vi "Version_2.0_Single_Column_Code.vi"() -> ()   [LabVIEW 2020] (continued)
                                frame True {
                                n9494 = local read "VISA Refnum in\nfor Pump"() -> (w9876:refnum<visa-resource-name>)
                                n9495 = call "HardStopCurrentProcess (SubVI).vi"("VISA Refnum in"=w9876) -> ()  [unwired: 11 in]
                                }
                                }
                                n9496 = call "ProcessCompletionWaiter (SubVI).vi"("VISA Refnum in"=w9875) -> ()  [unwired: 11 in]
                                }
                                frame #6 {
                                n9497 = local read "VISA Refnum in\nfor Pump"() -> (w9881:refnum<visa-resource-name>)
                                n9498 = local read "Volume of Syringe"() -> (w9878:dbl)
                                n9499 = call "GoToAbsolutePosition(SubVI).vi"("Absolute Volume Position in Syringe (in ul)"=0.0, "Volume of Syringe"=w9878, "Resolution of Pumping"=T2."Standard Pumping", "Flow Rate (ul/min)"=150.0, "VISA Refnum in"=w9881) -> ()  [unwired: 6 in, 1 out]
                                }
                                frame #7 {
                                n9500 = local read "Stopper that ends \nthe main loops"() -> (w9882:bool)
                                n9501 = local read "VISA Refnum in\nfor Pump"() -> (w9883:refnum<visa-resource-name>)
                                n9502 = case shown="True" w9882 {
                                frame False {
                                }
                                frame True {
                                n9503 = local read "VISA Refnum in\nfor Pump"() -> (w9884:refnum<visa-resource-name>)
                                n9504 = call "HardStopCurrentProcess (SubVI).vi"("VISA Refnum in"=w9884) -> ()  [unwired: 11 in]
                                }
                                }
                                n9505 = call "ProcessCompletionWaiter (SubVI).vi"("VISA Refnum in"=w9883) -> ()  [unwired: 11 in]
                                }
                              }
                            }
                          }
                        }
                      }
                      frame #4 {
                        n9506 = local read "VISA Refnum in\nfor Pump"() -> (w9886:refnum<visa-resource-name>)
                        n9507 = local read "Port for \nC2-Elution"() -> (w9885:string)
                        n9508 = call "PortChanger (SubVI).vi"("Port Number"=w9885, "VISA Refnum in"=w9886) -> ()  [unwired: 10 in]
                      }
                      frame #5 {
                        n9509 = local read "VISA Refnum in\nfor Pump"() -> (w9887:refnum<visa-resource-name>)
                        n9510 = call "ProcessCompletionWaiter (SubVI).vi"("VISA Refnum in"=w9887) -> ()  [unwired: 11 in]
                      }
                      frame #6 {
                        n9511 = local read "Buffer-C2 PickUp \nFlow Rate (ul/min)"() -> (w9891:dbl)
                        n9512 = local read "Buffer-C2 Pumping\nResolution"() -> (w9890:T2)
                        n9513 = local read "VISA Refnum in\nfor Pump"() -> (w9893:refnum<visa-resource-name>)
                        n9514 = local read "Buffer-C2 Volume \nto be Pumped"() -> (w9889:dbl)
                        n9515 = local read "Volume of Syringe"() -> (w9892:dbl)
                        n9516 = call "RPickUp(SubVI).vi"("Volume to be picked up"=w9889, "Volume of Syringe"=w9892, "Resolution of PickUP"=w9890, "PickUp Flow Rate (ul/min)"=w9891, "VISA Refnum in"=w9893) -> ()  [unwired: 6 in, 1 out]
                        n9517 = local write "SEC On"(TRUE ("SEC On")) -> ()
                      }
                      frame #7 {
                        n9518 = local read "Stopper that ends \nthe main loops"() -> (w9894:bool)
                        n9519 = local read "VISA Refnum in\nfor Pump"() -> (w9895:refnum<visa-resource-name>)
                        n9520 = case shown="True" w9894 {
                          frame False {
                          }
                          frame True {
                            n9521 = local read "VISA Refnum in\nfor Pump"() -> (w9896:refnum<visa-resource-name>)
                            n9522 = call "HardStopCurrentProcess (SubVI).vi"("VISA Refnum in"=w9896) -> ()  [unwired: 11 in]
                          }
                        }
                        n9523 = call "ProcessCompletionWaiter (SubVI).vi"("VISA Refnum in"=w9895) -> ()  [unwired: 11 in]
                      }
                      frame #8 {
                        # "Reads the initial Plunger Position for computing the volume dispensed"
                        n9524 = local read "VISA Refnum in\nfor Pump"() -> (w9898:refnum<visa-resource-name>)
                        n9525 = call "AbsolutePlungerPosition (SubVI).vi"("VISA Refnum in"=w9898) -> ("Plunger Position"=w9897:i32)  [unwired: 10 in]
                        n9526 = local write "Initial Plunger Position"(w9897) -> ()
                      }
                      frame #9 {
                        # "Switch to Port-10"
                        # "Port-10 of the pump is conncted to column-2 of chip"
                        n9527 = local read "VISA Refnum in\nfor Pump"() -> (w9900:refnum<visa-resource-name>)
                        n9528 = call "PortChanger (SubVI).vi"("Port Number"="10", "VISA Refnum in"=w9900) -> ()  [unwired: 10 in]
                      }
                      frame #10 {
                        n9529 = local read "Stopper that ends \nthe main loops"() -> (w9901:bool)
                        n9530 = local read "VISA Refnum in\nfor Pump"() -> (w9902:refnum<visa-resource-name>)
                        n9531 = call "ProcessCompletionWaiter (SubVI).vi"("VISA Refnum in"=w9902) -> ()  [unwired: 11 in]
                        n9532 = case shown="True" w9901 {
                          frame False {
                          }
                          frame True {
                            n9533 = local read "VISA Refnum in\nfor Pump"() -> (w9903:refnum<visa-resource-name>)
                            n9534 = call "HardStopCurrentProcess (SubVI).vi"("VISA Refnum in"=w9903) -> ()  [unwired: 11 in]
                          }
                        }
                      }
                      frame #11 {
                        # "Keeps the AMF valve after column-1 open and valve after column-2 closed"
                        n9535 = local read "Buffer-C2 Dispense\nFlow Rate (ul/min)"() -> (w9916:dbl)
                        n9536 = local read "Buffer-C2 Pumping\nResolution"() -> (w9915:T2)
                        n9537 = local read "VISA Refnum in\nfor Pump"() -> (w9918:refnum<visa-resource-name>)
                        n9538 = local write "Pause Data Collection"(FALSE ("Pause Data Collection")) -> ()
                        n9539 = local read "Volume of Syringe"() -> (w9917:dbl)
                        n9540 = call "GoToAbsolutePosition(SubVI).vi"("Absolute Volume Position in Syringe (in ul)"=0.0 ("Volume to be Dispensed"), "Volume of Syringe"=w9917, "Resolution of Pumping"=w9915, "Flow Rate (ul/min)"=w9916, "VISA Refnum in"=w9918) -> ()  [unwired: 6 in, 1 out]
                        n9541 = local write "Valve V1 Open"(FALSE ("Valve V1 Open")) -> ()
                        n9542 = local write "Valve V2 Open"(TRUE ("Valve V2 Open")) -> ()
                        n9543 = local write "Valve V3 Open"(TRUE ("Valve V3 Open")) -> ()
                        n9544 = local write "Valve V4 Open"(FALSE ("Valve V4 Open")) -> ()
                        n9545 = local write "External Valve \nOpen"(TRUE ("External Valve \nOpen")) -> ()
                        n9546 = local write "Valve V8 Open"(FALSE ("Valve V8 Open")) -> ()
                        n9547 = local write "Valve V5 Open"(FALSE ("Valve V5 Open")) -> ()
                        n9548 = local write "Valve V6 Open"(FALSE ("Valve V6 Open")) -> ()
                        n9549 = local write "Valve V7 Open"(FALSE ("Valve V7 Open")) -> ()
                      }
                      frame #12 {
                        n9550 = local read "Initial Plunger Position"() -> (w9922:dbl)
                        n9551 = local read "Buffer-C2 Pumping\nResolution"() -> (w9921:T2)
                        n9552 = local read "VISA Refnum in\nfor Pump"() -> (w9923:refnum<visa-resource-name>)
                        n9553 = local read "Volume of Syringe"() -> (w9920:dbl)
                        n9554 = while {
                          tunnel: w9922 -> [w9929]
                          tunnel: w9923 -> [w9928]
                          tunnel: w9921 -> [w9927]
                          tunnel: w9920 -> [w9926]
                          stop <- w9924 stop-if-true
                          n9555 = Wait (ms)(milliseconds to wait=u32 100) -> ()  [unwired: 1 out]
                          n9556 = stacked-sequence {
                            tunnel: w9929 -> [w9935 _]
                            tunnel: w9928 -> [w9934 w9961]
                            tunnel: w9927 -> [w9933 _]
                            tunnel: w9926 -> [w9932 _]
                            tunnel: [_ w9957] -> w9924
                            frame #0 {
                              n9557 = call "AbsolutePlungerPosition (SubVI).vi"("VISA Refnum in"=w9934) -> ("Plunger Position"=w9931:i32)  [unwired: 10 in]
                              n9558 = case shown="\"Standard Pumping\", Default" w9933 {
                                tunnel: w9935 -> [w9940 w9949]
                                tunnel: w9931 -> [w9941 w9948]
                                tunnel: [w9939 w9946] -> w9930
                                tunnel: w9932 -> [w9938 w9947]
                                frame "Standard Pumping", Default {
                                n9559 = Subtract(x=w9940, y=w9941) -> (x-y=w9937:dbl)
                                n9560 = Absolute Value(x=w9937) -> (abs(x)=w9936:dbl)
                                n9561 = Multiply(x=w9936, y=w9938) -> (x*y=w9943:dbl)
                                n9562 = Divide(x=w9943, y=3000.0) -> (x/y=w9939:dbl)
                                }
                                frame "High Resolution Pumping" {
                                n9563 = Subtract(x=w9949, y=w9948) -> (x-y=w9945:dbl)
                                n9564 = Absolute Value(x=w9945) -> (abs(x)=w9944:dbl)
                                n9565 = Multiply(x=w9944, y=w9947) -> (x*y=w9951:dbl)
                                n9566 = Divide(x=w9951, y=24000.0) -> (x/y=w9946:dbl)
                                }
                              }
                              n9567 = local write "Volume being Injected \nin this process"(w9930) -> ()
                            }
                            frame #1 {
                              n9568 = local read "Stopper that ends \nthe main loops"() -> (w9958:bool)
                              n9569 = local read "Divert Buffer-C \ninto Column-2"() -> (w9959:bool)
                              n9570 = local read "Volume being Injected \nin this process"() -> (w9956:dbl)
                              n9571 = call "LSPOneStatus (SubVI).vi"("VISA Refnum in"=w9961) -> ("read buffer"=w9963:string)  [unwired: 10 in]
                              n9572 = call <vilib>:"Trim Whitespace.vi"("string"=w9963) -> ("trimmed string"=w9962:string)  [unwired: 1 in]
                              n9573 = Equal?(x=w9962, y="/0`\u0003") -> (x = y?=w9960:bool)
                              n9574 = Or(x=w9959, y=w9958) -> (x .or. y?=w9954:bool)
                              n9575 = Greater Or Equal?(x=w9956, y=2.0) -> (x >= y?=w9953:bool)
                              n9576 = Or(x=w9954, y=w9953) -> (x .or. y?=w9952:bool)
                              n9577 = Or(x=w9960, y=w9952) -> (x .or. y?=w9957:bool)
                            }
                          }
                        }
                        n9578 = local read "Stopper that ends \nthe main loops"() -> (w9919:bool)
                        n9579 = case shown="True" w9919 {
                          frame False {
                          }
                          frame True {
                            n9580 = local read "VISA Refnum in\nfor Pump"() -> (w9965:refnum<visa-resource-name>)
                            n9581 = call "HardStopCurrentProcess (SubVI).vi"("VISA Refnum in"=w9965) -> ()  [unwired: 11 in]
                          }
                        }
                      }
                      frame #13 {
                        # "Keeps the on-chip valves V4, V5 and V7 open"
                        # "Keeps the AMF valve after column-1 closed and valve after column-2 open"
                        n9582 = local write "Divert Buffer-C \ninto Column-2"(FALSE ("Divert Buffer-C \ninto Column-2")) -> ()
                        n9583 = local write "Valve V3 Open"(TRUE ("Valve V3 Open")) -> ()
                        n9584 = local write "Valve V2 Open"(FALSE ("Valve V2 Open")) -> ()
                        n9585 = local write "Valve V1 Open"(FALSE ("Valve V1 Open")) -> ()
                        n9586 = local write "Valve V4 Open"(TRUE ("Valve V4 Open")) -> ()
                        n9587 = local write "External Valve \nOpen"(FALSE ("External Valve \nOpen")) -> ()
                        n9588 = local write "Valve V5 Open"(TRUE ("Valve V5 Open")) -> ()
                        n9589 = local write "Valve V6 Open"(FALSE ("Valve V6 Open")) -> ()
                        n9590 = local write "Valve V8 Open"(FALSE ("Valve V8 Open")) -> ()
                        n9591 = local write "Valve V7 Open"(TRUE ("Valve V7 Open")) -> ()
                      }
                      frame #14 {
                        n9592 = local read "Initial Plunger Position"() -> (w9979:dbl)
                        n9593 = local read "Buffer-C2 Pumping\nResolution"() -> (w9978:T2)
                        n9594 = local read "VISA Refnum in\nfor Pump"() -> (w9980:refnum<visa-resource-name>)
                        n9595 = local read "Volume of Syringe"() -> (w9977:dbl)
                        n9596 = while {
                          tunnel: w9979 -> [w9986]
                          tunnel: w9980 -> [w9985]
                          tunnel: w9978 -> [w9984]
                          tunnel: w9977 -> [w9983]
                          stop <- w9981 stop-if-true
                          n9597 = Wait (ms)(milliseconds to wait=u32 100) -> ()  [unwired: 1 out]
                          n9598 = stacked-sequence {
                            tunnel: w9986 -> [w9992 _]
                            tunnel: w9985 -> [w9991 w10014]
                            tunnel: w9984 -> [w9990 _]
                            tunnel: w9983 -> [w9989 _]
                            tunnel: [_ w10012] -> w9981
                            frame #0 {
                              n9599 = call "AbsolutePlungerPosition (SubVI).vi"("VISA Refnum in"=w9991) -> ("Plunger Position"=w9988:i32)  [unwired: 10 in]
                              n9600 = case shown="\"Standard Pumping\", Default" w9990 {
                                tunnel: w9992 -> [w9997 w10006]
                                tunnel: w9988 -> [w9998 w10005]
                                tunnel: [w9996 w10003] -> w9987
                                tunnel: w9989 -> [w9995 w10004]
                                frame "Standard Pumping", Default {
                                n9601 = Subtract(x=w9997, y=w9998) -> (x-y=w9994:dbl)
                                n9602 = Absolute Value(x=w9994) -> (abs(x)=w9993:dbl)
                                n9603 = Multiply(x=w9993, y=w9995) -> (x*y=w10000:dbl)
                                n9604 = Divide(x=w10000, y=3000.0) -> (x/y=w9996:dbl)
                                }
                                frame "High Resolution Pumping" {
                                n9605 = Subtract(x=w10006, y=w10005) -> (x-y=w10002:dbl)
                                n9606 = Absolute Value(x=w10002) -> (abs(x)=w10001:dbl)
                                n9607 = Multiply(x=w10001, y=w10004) -> (x*y=w10008:dbl)
                                n9608 = Divide(x=w10008, y=24000.0) -> (x/y=w10003:dbl)
                                }
                              }
                              n9609 = local write "Volume being Injected \nin this process"(w9987) -> ()
                            }
                            frame #1 {
                              n9610 = call "LSPOneStatus (SubVI).vi"("VISA Refnum in"=w10014) -> ("read buffer"=w10016:string)  [unwired: 10 in]
                              n9611 = call <vilib>:"Trim Whitespace.vi"("string"=w10016) -> ("trimmed string"=w10015:string)  [unwired: 1 in]
                              n9612 = Equal?(x=w10015, y="/0`\u0003") -> (x = y?=w10013:bool)
                              n9613 = local read "Stopper that ends \nthe main loops"() -> (w10010:bool)
                              n9614 = local read "Divert Sample \nonto Grid"() -> (w10011:bool)
                              n9615 = Or(x=w10011, y=w10010) -> (x .or. y?=w10009:bool)
                              n9616 = Or(x=w10013, y=w10009) -> (x .or. y?=w10012:bool)
                            }
                          }
                        }
                        n9617 = local read "Stopper that ends \nthe main loops"() -> (w9976:bool)
                        n9618 = case shown="True" w9976 {
                          frame False {
                          }
                          frame True {
                            n9619 = local read "VISA Refnum in\nfor Pump"() -> (w10018:refnum<visa-resource-name>)
                            n9620 = call "HardStopCurrentProcess (SubVI).vi"("VISA Refnum in"=w10018) -> ()  [unwired: 11 in]
                          }
                        }
                      }
                      frame #15 {
                        n9621 = local read "Volume being Injected \nin this process"() -> (w10021:dbl)
                        n9622 = local read "VISA Refnum in\nfor Pump"() -> (w10023:refnum<visa-resource-name>)
                        n9623 = call "AbsolutePlungerPosition (SubVI).vi"("VISA Refnum in"=w10023) -> ("Plunger Position"=w10022:i32)  [unwired: 10 in]
                        n9624 = local write "Pause Data Collection"(TRUE) -> ()
                        n9625 = local write "True Volume being \ninjected in this\nprocess"(w10021) -> ()
                        n9626 = local write "Position\nNow"(w10022) -> ()
                        n9627 = Wait (ms)(milliseconds to wait=u32 500) -> ()  [unwired: 1 out]
                      }
                      frame #16 {
                        # "Sample Deposition onto EM-Grid"
                        n9628 = local read "Divert Sample \nonto Grid"() -> (w10024:bool)
                        n9629 = case shown="True" w10024 {
                          frame False {
                          }
                          frame True {
                            n9630 = stacked-sequence {
                              frame #0 {
                                # "Discard the initial volume of fluid that is present in the channel prior to detection"
                                n9631 = local read "Buffer-C2 Pumping\nResolution"() -> (w10037:T2)
                                n9632 = local read "Initial Plunger Position"() -> (w10036:dbl)
                                n9633 = local read "VISA Refnum in\nfor Pump"() -> (w10038:refnum<visa-resource-name>)
                                n9634 = local read "Position\nNow"() -> (w10034:dbl)
                                n9635 = local read "Volume of Syringe"() -> (w10035:dbl)
                                n9636 = local write "Pause Data Collection"(FALSE) -> ()
                                n9637 = while {
                                tunnel: w10038 -> [w10048]
                                tunnel: w10037 -> [w10047]
                                tunnel: w10036 -> [w10043]
                                tunnel: w10035 -> [w10046]
                                tunnel: w10034 -> [w10042]
                                stop <- w10044 stop-if-true
                                n9638 = stacked-sequence {
                                tunnel: w10048 -> [w10054 w10076 w10108]
                                tunnel: w10047 -> [w10053 w10075 _]
                                tunnel: w10043 -> [w10051 _ _]
                                tunnel: w10046 -> [w10050 w10073 _]
                                tunnel: [_ _ w10102] -> w10044
                                tunnel: w10042 -> [_ w10071 _]
                                frame #0 {
                                # "From here on 'True Volume being injected \nin this process' represents the true total \nvolume in this process"
                                n9639 = call "AbsolutePlungerPosition (SubVI).vi"("VISA Refnum in"=w10054) -> ("Plunger Position"=w10052:i32)  [unwired: 10 in]
                                n9640 = case shown="..\"Standard Pumping\"" w10053 {
                                tunnel: w10052 -> [w10062 w10070]
                                tunnel: w10051 -> [w10061 w10069]
                                tunnel: w10050 -> [w10058 w10066]
                                tunnel: [w10055 w10063] -> w10049
                                frame .."Standard Pumping" {
                                n9641 = Subtract(x=w10062, y=w10061) -> (x-y=w10060:dbl)
                                n9642 = Absolute Value(x=w10060) -> (abs(x)=w10059:dbl)
                                n9643 = Multiply(x=w10059, y=w10058) -> (x*y=w10057:dbl)
                                n9644 = Divide(x=w10057, y=3000.0) -> (x/y=w10055:dbl)
                                }
                                frame "High Resolution Pumping".. {
                                n9645 = Subtract(x=w10070, y=w10069) -> (x-y=w10068:dbl)
                                n9646 = Absolute Value(x=w10068) -> (abs(x)=w10067:dbl)
                                n9647 = Multiply(x=w10067, y=w10066) -> (x*y=w10065:dbl)
                                n9648 = Divide(x=w10065, y=24000.0) -> (x/y=w10063:dbl)
                                }
                                }
                                n9649 = local write "True Volume being \ninjected in this\nprocess"(w10049) -> ()
                                }
                                frame #1 {
                                # "From here on 'Volume being injected \nin this process' represents the volume \nin this sub process"
                                n9650 = call "AbsolutePlungerPosition (SubVI).vi"("VISA Refnum in"=w10076) -> ("Plunger Position"=w10074:i32)  [unwired: 10 in]
                                n9651 = case shown="..\"Standard Pumping\"" w10075 {
                                tunnel: w10074 -> [w10084 w10092]
                                tunnel: w10071 -> [w10083 w10091]
                                tunnel: w10073 -> [w10080 w10088]
                                tunnel: [w10077 w10085] -> w10072
                                frame .."Standard Pumping" {
                                n9652 = Subtract(x=w10084, y=w10083) -> (x-y=w10082:dbl)
                                n9653 = Absolute Value(x=w10082) -> (abs(x)=w10081:dbl)
                                n9654 = Multiply(x=w10081, y=w10080) -> (x*y=w10079:dbl)
                                n9655 = Divide(x=w10079, y=3000.0) -> (x/y=w10077:dbl)
                                }
                                frame "High Resolution Pumping".. {
                                n9656 = Subtract(x=w10092, y=w10091) -> (x-y=w10090:dbl)
                                n9657 = Absolute Value(x=w10090) -> (abs(x)=w10089:dbl)
                                n9658 = Multiply(x=w10089, y=w10088) -> (x*y=w10087:dbl)
                                n9659 = Divide(x=w10087, y=24000.0) -> (x/y=w10085:dbl)
                                }
                                }
                                n9660 = local write "Volume being Injected \nin this process"(w10072) -> ()
                                }
                                frame #2 {
                                n9661 = local read "Discard Volume"() -> (w10096:dbl)
                                n9662 = local read "Discard fluid \nprior to 1st \ndeposition"() -> (w10101:bool)
                                n9663 = local read "Volume being Injected \nin this process"() -> (w10100:dbl)
                                n9664 = Greater Or Equal?(x=w10100, y=w10096) -> (x >= y?=w10098:bool)
                                n9665 = call "AbsolutePlungerPositionStatus (SubVI).vi"("VISA Refnum in"=w10108) -> ("read buffer"=w10107:string)  [unwired: 10 in]
                                n9666 = local read "Stop for End of \nExperiment \nand Data Writing"() -> (w10095:bool)
                                n9667 = call <vilib>:"Trim Whitespace.vi"("string"=w10107) -> ("trimmed string"=w10106:string)  [unwired: 1 in]
                                n9668 = Not(x=w10101) -> (.not. x?=w10099:bool)
                                n9669 = Equal?(x=w10106, y="/0`\u0003") -> (x = y?=w10104:bool)
                                n9670 = Or(x=w10099, y=w10098) -> (x .or. y?=w10097:bool)
                                n9671 = local read "Re-SEC"() -> (w10094:bool)
                                n9672 = Or(x=w10095, y=w10094) -> (x .or. y?=w10093:bool)
                                n9673 = Or(x=w10097, y=w10093) -> (x .or. y?=w10103:bool)
                                n9674 = Or(x=w10104, y=w10103) -> (x .or. y?=w10102:bool)
                                }
                                }
                                n9675 = Wait (ms)(milliseconds to wait=u32 100) -> ()  [unwired: 1 out]
                                }
                                n9676 = local write "Valve V4 Open"(TRUE ("Valve V4 Open")) -> ()
                                n9677 = local write "Valve V3 Open"(TRUE ("Valve V3 Open")) -> ()
                                n9678 = local write "Valve V2 Open"(FALSE ("Valve V2 Open")) -> ()
                                n9679 = local write "Valve V1 Open"(FALSE ("Valve V1 Open")) -> ()
                                n9680 = local write "External Valve \nOpen"(FALSE ("External Valve \nOpen")) -> ()
                                n9681 = local write "Valve V5 Open"(TRUE ("Valve V5 Open")) -> ()
                                n9682 = local write "Valve V6 Open"(TRUE ("Valve V6 Open")) -> ()
                                n9683 = local write "Valve V8 Open"(FALSE ("Valve V8 Open")) -> ()
                                n9684 = local write "Valve V7 Open"(FALSE ("Valve V7 Open")) -> ()
                                n9685 = local write "Volume being Injected \nin this process"(0.0) -> ()
                              }
                              frame #1 {
                                # "Keeps the on-chip valve V1, V2 and V3 closed,\nHalts also deposition onto the grid\nand waits for the 1st redeposit command. Once the command is issued\nit starts pumpoing and moves onto the next frame"
                                n9686 = stacked-sequence {
                                frame #0 {
                                n9687 = local write "Valve V5 Open"(FALSE ("Valve V5 Open")) -> ()
                                n9688 = local write "Valve V1 Open"(FALSE ("Valve V1 Open")) -> ()
                                n9689 = local read "VISA Refnum in\nfor Pump"() -> (w10120:refnum<visa-resource-name>)
                                n9690 = local write "Valve V2 Open"(FALSE ("Valve V2 Open")) -> ()
                                n9691 = local write "Valve V6 Open"(FALSE ("Valve V6 Open")) -> ()
                                n9692 = local write "Re-deposit Sample\nonto Grid"(FALSE ("Redeposit Sample\nonto Grid")) -> ()
                                n9693 = local write "Pause Data Collection"(TRUE ("Pause Data Collection")) -> ()
                                n9694 = call "HardStopCurrentProcess (SubVI).vi"("VISA Refnum in"=w10120) -> ()  [unwired: 11 in]
                                n9695 = local write "Valve V7 Open"(FALSE ("Valve V7 Open")) -> ()
                                n9696 = local write "Valve V3 Open"(FALSE ("Valve V3 Open")) -> ()
                                n9697 = local write "External Valve \nOpen"(FALSE ("External Valve \nOpen")) -> ()
                                n9698 = local write "Valve V4 Open"(FALSE ("Valve V4 Open")) -> ()
                                n9699 = local write "Valve V8 Open"(FALSE ("Valve V8 Open")) -> ()
                                }
                                frame #1 {
                                n9700 = while {
                                stop <- w10126 stop-if-true
                                n9701 = local read "Stop for End of \nExperiment \nand Data Writing"() -> (w10124:bool)
                                n9702 = local read "Re-SEC"() -> (w10125:bool)
                                n9703 = local read "Re-deposit Sample\nonto Grid"() -> (w10127:bool)
                                n9704 = Or(x=w10124, y=w10125) -> (x .or. y?=w10123:bool)
                                n9705 = Or(x=w10127, y=w10123) -> (x .or. y?=w10126:bool)
                                }
                                n9706 = local write "Discard fluid \nprior to 1st \ndeposition"(FALSE ("Discard fluid \nprior to 1st \ndeposition")) -> ()
                                n9707 = One Button Dialog(message="Do you want to deposit sample on another grid? If yes, turn on 'Re-deposit Sample onto Grid'. Else turn on Re-SEC to do SEC again or STOP to end the experiment") -> ()  [unwired: 1 in, 1 out]
                                }
                                frame #2 {
                                n9708 = local write "Valve V6 Open"(TRUE ("Valve V3 Open")) -> ()
                                n9709 = local write "Valve V4 Open"(TRUE ("Valve V1 Open")) -> ()
                                n9710 = local write "Valve V5 Open"(TRUE ("Valve V2 Open")) -> ()
                                n9711 = local write "Valve V3 Open"(TRUE ("Valve V3 Open")) -> ()
                                n9712 = local write "Valve V7 Open"(FALSE ("Valve V7 Open")) -> ()
                                }
                                frame #3 {
                                n9713 = local read "Re-deposit Sample\nonto Grid"() -> (w10133:bool)
                                n9714 = case shown="True" w10133 {
                                frame False {
                                n9715 = local write "Suction On/Off"(FALSE ("Suction On/Off")) -> ()
                                }
                                frame True {
                                n9716 = stacked-sequence {
                                frame #0 {
                                n9717 = local read "VISA Refnum in\nfor Pump"() -> (w10136:refnum<visa-resource-name>)
                                n9718 = call "AbsolutePlungerPosition (SubVI).vi"("VISA Refnum in"=w10136) -> ("Plunger Position"=w10135:i32)  [unwired: 10 in]
                                n9719 = local write "Position\nNow"(w10135) -> ()
                                }
                                frame #1 {
                                n9720 = local read "Buffer-C2 Pumping\nResolution"() -> (w10138:T2)
                                n9721 = case shown="\"Standard Pumping\", Default" w10138 {
                                tunnel: [w10139 w10150] -> w10137
                                frame "Standard Pumping", Default {
                                n9722 = local read "Buffer-C2 Volume \nto be Pumped"() -> (w10142:dbl)
                                n9723 = local read "Volume of Syringe"() -> (w10145:dbl)
                                n9724 = local read "Initial Plunger Position"() -> (w10149:dbl)
                                n9725 = local read "Position\nNow"() -> (w10148:dbl)
                                n9726 = Subtract(x=w10149, y=w10148) -> (x-y=w10147:dbl)
                                n9727 = Absolute Value(x=w10147) -> (abs(x)=w10146:dbl)
                                n9728 = Multiply(x=w10146, y=w10145) -> (x*y=w10144:dbl)
                                n9729 = Divide(x=w10144, y=3000.0) -> (x/y=w10141:dbl)
                                n9730 = Subtract(x=w10141, y=w10142) -> (x-y=w10140:dbl)
                                n9731 = Absolute Value(x=w10140) -> (abs(x)=w10139:dbl)
                                }
                                frame "High Resolution Pumping" {
                                n9732 = local read "Buffer-C2 Volume \nto be Pumped"() -> (w10153:dbl)
                                n9733 = local read "Volume of Syringe"() -> (w10156:dbl)
                                n9734 = local read "Initial Plunger Position"() -> (w10160:dbl)
                                n9735 = local read "Position\nNow"() -> (w10159:dbl)
                                n9736 = Subtract(x=w10160, y=w10159) -> (x-y=w10158:dbl)
                                n9737 = Absolute Value(x=w10158) -> (abs(x)=w10157:dbl)
                                n9738 = Multiply(x=w10157, y=w10156) -> (x*y=w10155:dbl)
                                n9739 = Divide(x=w10155, y=24000.0) -> (x/y=w10152:dbl)
                                n9740 = Subtract(x=w10152, y=w10153) -> (x-y=w10151:dbl)
                                n9741 = Absolute Value(x=w10151) -> (abs(x)=w10150:dbl)
                                }
                                }
                                n9742 = local write "Buffer-C Volume\nleft to be Pumped"(w10137) -> ()
                                }
                                frame #2 {
                                n9743 = local read "Buffer-C2 Dispense\nFlow Rate (ul/min)"() -> (w10164:dbl)
                                n9744 = local read "Buffer-C2 Pumping\nResolution"() -> (w10163:T2)
                                n9745 = local read "VISA Refnum in\nfor Pump"() -> (w10166:refnum<visa-resource-name>)
                                n9746 = local read "Volume of Syringe"() -> (w10165:dbl)
                                n9747 = call "GoToAbsolutePosition(SubVI).vi"("Absolute Volume Position in Syringe (in ul)"=0.0, "Volume of Syringe"=w10165, "Resolution of Pumping"=w10163, "Flow Rate (ul/min)"=w10164, "VISA Refnum in"=w10166) -> ()  [unwired: 6 in, 1 out]
                                n9748 = local write "Suction On/Off"(FALSE ("Suction On/Off")) -> ()
                                }
                                }
                                }
                                }
                                }
                                frame #4 {
                                n9749 = local read "Stop for End of \nExperiment \nand Data Writing"() -> (w10169:bool)
                                n9750 = local read "Re-SEC"() -> (w10168:bool)
                                n9751 = Or(x=w10169, y=w10168) -> (x .or. y?=w10167:bool)
                                n9752 = case shown="True" w10167 {
                                frame False {
                                }
                                frame True {
                                n9753 = local read "VISA Refnum in\nfor Pump"() -> (w10170:refnum<visa-resource-name>)
                                n9754 = call "HardStopCurrentProcess (SubVI).vi"("VISA Refnum in"=w10170) -> ()  [unwired: 11 in]
                                }
                                }
                                }
                                }
                              }
                              frame #2 {
                                # "Keeps the on-chip valve V1, V2 Open and V3 closed"
                                n9755 = while {
                                stop <- w10176 stop-if-true
                                n9756 = local read "Suction On/Off"() -> (w10177:bool)
                                n9757 = case shown="True" w10177 {
                                frame False {
                                n9758 = local read "Buffer-C2 Pumping\nResolution"() -> (w10183:T2)
                                n9759 = local read "Initial Plunger Position"() -> (w10182:dbl)
                                n9760 = local read "VISA Refnum in\nfor Pump"() -> (w10184:refnum<visa-resource-name>)
                                n9761 = local read "Position\nNow"() -> (w10180:dbl)
                                n9762 = local read "Volume of Syringe"() -> (w10181:dbl)
                                n9763 = local write "Volume being Injected \nin this process"(0.0) -> ()
                                n9764 = local write "Pause Data Collection"(FALSE) -> ()
                                n9765 = while {
                                tunnel: w10184 -> [w10191]
                                tunnel: w10183 -> [w10190]
                                tunnel: w10182 -> [w10186]
                                tunnel: w10181 -> [w10189]
                                tunnel: w10180 -> [w10185]
                                stop <- w10187 stop-if-true
                                n9766 = stacked-sequence {
                                tunnel: w10191 -> [w10197 w10219 w10246]
                                tunnel: w10190 -> [w10196 w10218 _]
                                tunnel: w10186 -> [w10194 _ _]
                                tunnel: w10189 -> [w10193 w10216 _]
                                tunnel: [_ _ w10239] -> w10187
                                tunnel: w10185 -> [_ w10214 _]
                                frame #0 {
                                # "From here on 'True Volume being injected \nin this process' represents the true total \nvolume in this process"
                                n9767 = call "AbsolutePlungerPosition (SubVI).vi"("VISA Refnum in"=w10197) -> ("Plunger Position"=w10195:i32)  [unwired: 10 in]
                                n9768 = case shown="..\"Standard Pumping\"" w10196 {
                                tunnel: w10195 -> [w10205 w10213]
                                tunnel: w10194 -> [w10204 w10212]
                                tunnel: w10193 -> [w10201 w10209]
                                tunnel: [w10198 w10206] -> w10192
                                frame .."Standard Pumping" {
                                n9769 = Subtract(x=w10205, y=w10204) -> (x-y=w10203:dbl)
                                n9770 = Absolute Value(x=w10203) -> (abs(x)=w10202:dbl)
                                n9771 = Multiply(x=w10202, y=w10201) -> (x*y=w10200:dbl)
                                n9772 = Divide(x=w10200, y=3000.0) -> (x/y=w10198:dbl)
                                }
                                frame "High Resolution Pumping".. {
                                n9773 = Subtract(x=w10213, y=w10212) -> (x-y=w10211:dbl)
                                n9774 = Absolute Value(x=w10211) -> (abs(x)=w10210:dbl)
                                n9775 = Multiply(x=w10210, y=w10209) -> (x*y=w10208:dbl)
                                n9776 = Divide(x=w10208, y=24000.0) -> (x/y=w10206:dbl)
                                }
                                }
                                n9777 = local write "True Volume being \ninjected in this\nprocess"(w10192) -> ()
                                }
                                frame #1 {
                                # "From here on 'Volume being injected \nin this process' represents the volume \nin this sub process"
                                n9778 = call "AbsolutePlungerPosition (SubVI).vi"("VISA Refnum in"=w10219) -> ("Plunger Position"=w10217:i32)  [unwired: 10 in]
                                n9779 = case shown="\"High Resolution Pumping\".." w10218 {
                                tunnel: w10217 -> [w10227 w10235]
                                tunnel: w10214 -> [w10226 w10234]
                                tunnel: w10216 -> [w10223 w10231]
                                tunnel: [w10220 w10228] -> w10215
                                frame .."Standard Pumping" {
                                n9780 = Subtract(x=w10227, y=w10226) -> (x-y=w10225:dbl)
                                n9781 = Absolute Value(x=w10225) -> (abs(x)=w10224:dbl)
                                n9782 = Multiply(x=w10224, y=w10223) -> (x*y=w10222:dbl)
                                n9783 = Divide(x=w10222, y=3000.0) -> (x/y=w10220:dbl)
                                }
                                frame "High Resolution Pumping".. {
                                n9784 = Subtract(x=w10235, y=w10234) -> (x-y=w10233:dbl)
                                n9785 = Absolute Value(x=w10233) -> (abs(x)=w10232:dbl)
                                n9786 = Multiply(x=w10232, y=w10231) -> (x*y=w10230:dbl)
                                n9787 = Divide(x=w10230, y=24000.0) -> (x/y=w10228:dbl)
                                }
                                }
                                n9788 = local write "Volume being Injected \nin this process"(w10215) -> ()
                                }
                                frame #2 {
                                n9789 = local read "Stop for End of \nExperiment \nand Data Writing"() -> (w10238:bool)
                                n9790 = local read "Re-SEC"() -> (w10237:bool)
                                n9791 = local read "Suction On/Off"() -> (w10242:bool)
                                n9792 = call "AbsolutePlungerPositionStatus (SubVI).vi"("VISA Refnum in"=w10246) -> ("read buffer"=w10245:string)  [unwired: 10 in]
                                n9793 = call <vilib>:"Trim Whitespace.vi"("string"=w10245) -> ("trimmed string"=w10244:string)  [unwired: 1 in]
                                n9794 = Equal?(x=w10244, y="/0`\u0003") -> (x = y?=w10241:bool)
                                n9795 = Or(x=w10238, y=w10237) -> (x .or. y?=w10236:bool)
                                n9796 = Or(x=w10242, y=w10236) -> (x .or. y?=w10240:bool)
                                n9797 = Or(x=w10241, y=w10240) -> (x .or. y?=w10239:bool)
                                }
                                }
                                n9798 = Wait (ms)(milliseconds to wait=u32 100) -> ()  [unwired: 1 out]
                                }
                                }
                                frame True {
                                n9799 = stacked-sequence {
                                frame #0 {
                                n9800 = local write "Valve V3 Open"(FALSE ("Valve V3 Open")) -> ()
                                n9801 = local read "Suction Pressure\nfor EM-grid \nDeposition (mbar)"() -> (w10253:sgl)
                                n9802 = local write "Valve V4 Open"(FALSE ("Valve V4 Open")) -> ()
                                n9803 = local read "VISA Refnum in\nfor Pump"() -> (w10256:refnum<visa-resource-name>)
                                n9804 = local write "Valve V5 Open"(FALSE ("Valve V1 Open")) -> ()
                                n9805 = local write "Suction pressure \nfor grid deposition"(w10253) -> ()
                                n9806 = local write "Re-deposit Sample\nonto Grid"(FALSE ("Redeposit Sample\nonto Grid")) -> ()
                                n9807 = local write "Pause Data Collection"(TRUE ("Pause Data Collection")) -> ()
                                n9808 = call "HardStopCurrentProcess (SubVI).vi"("VISA Refnum in"=w10256) -> ()  [unwired: 11 in]
                                n9809 = local write "Valve V6 Open"(TRUE ("Valve V2 Open")) -> ()
                                n9810 = local write "Valve V7 Open"(TRUE ("Valve V3 Open")) -> ()
                                n9811 = local write "External Valve \nOpen"(FALSE ("External Valve \nOpen")) -> ()
                                }
                                frame #1 {
                                n9812 = while {
                                stop <- w10259 stop-if-true
                                n9813 = local read "Stop for End of \nExperiment \nand Data Writing"() -> (w10260:bool)
                                n9814 = local read "Suction Pressure\nfor EM-grid \nDeposition (mbar)"() -> (w10257:sgl)
                                n9815 = call <vilib>:"fgt set pressure.vi"("pressure"=w10257, "pressureIndex"=u32 1) -> ()  [unwired: 9 in, 1 out]
                                n9816 = local read "Suction On/Off"() -> (w10262:bool)
                                n9817 = Not(x=w10262) -> (.not. x?=w10261:bool)
                                n9818 = Wait (ms)(milliseconds to wait=u32 100) -> ()  [unwired: 1 out]
                                n9819 = Or(x=w10261, y=w10260) -> (x .or. y?=w10259:bool)
                                }
                                }
                                frame #2 {
                                n9820 = for {
                                N: 2 -> [_]
                                n9821 = while {
                                stop <- w10272 stop-if-true
                                n9822 = local read "Stop for End of \nExperiment \nand Data Writing"() -> (w10268:bool)
                                n9823 = local read "Suction On/Off"() -> (w10270:bool)
                                n9824 = call <vilib>:"fgt set pressure.vi"("pressure"=sgl 0.0, "pressureIndex"=u32 1) -> ()  [unwired: 9 in, 1 out]
                                n9825 = Not(x=w10270) -> (.not. x?=w10269:bool)
                                n9826 = Wait (ms)(milliseconds to wait=u32 100) -> ()  [unwired: 1 out]
                                n9827 = Or(x=w10269, y=w10268) -> (x .or. y?=w10272:bool)
                                }
                                n9828 = Wait (ms)(milliseconds to wait=u32 400) -> ()  [unwired: 1 out]
                                }
                                }
                                frame #3 {
                                n9829 = local read "Automatic purging \nof capillary after \ngrid deposition"() -> (w10273:bool)
                                n9830 = case shown="True" w10273 {
                                frame False {
                                }
                                frame True {
                                n9831 = stacked-sequence {
                                frame #0 {
                                n9832 = local read "VISA Refnum in\nfor Pump"() -> (w10275:refnum<visa-resource-name>)
                                n9833 = call "AbsolutePlungerPosition (SubVI).vi"("VISA Refnum in"=w10275) -> ("Plunger Position"=w10274:i32)  [unwired: 10 in]
                                n9834 = local write "Position\nNow"(w10274) -> ()
                                }
                                frame #1 {
                                n9835 = local read "Buffer-C2 Pumping\nResolution"() -> (w10277:T2)
                                n9836 = case shown="\"Standard Pumping\", Default" w10277 {
                                tunnel: [w10278 w10289] -> w10276
                                frame "Standard Pumping", Default {
                                n9837 = local read "Buffer-C2 Volume \nto be Pumped"() -> (w10281:dbl)
                                n9838 = local read "Volume of Syringe"() -> (w10284:dbl)
                                n9839 = local read "Initial Plunger Position"() -> (w10288:dbl)
                                n9840 = local read "Position\nNow"() -> (w10287:dbl)
                                n9841 = Subtract(x=w10288, y=w10287) -> (x-y=w10286:dbl)
                                n9842 = Absolute Value(x=w10286) -> (abs(x)=w10285:dbl)
                                n9843 = Multiply(x=w10285, y=w10284) -> (x*y=w10283:dbl)
                                n9844 = Divide(x=w10283, y=3000.0) -> (x/y=w10280:dbl)
                                n9845 = Subtract(x=w10280, y=w10281) -> (x-y=w10279:dbl)
                                n9846 = Absolute Value(x=w10279) -> (abs(x)=w10278:dbl)
                                }
                                frame "High Resolution Pumping" {
                                n9847 = local read "Buffer-C2 Volume \nto be Pumped"() -> (w10292:dbl)
                                n9848 = local read "Volume of Syringe"() -> (w10295:dbl)
                                n9849 = local read "Initial Plunger Position"() -> (w10299:dbl)
                                n9850 = local read "Position\nNow"() -> (w10298:dbl)
                                n9851 = Subtract(x=w10299, y=w10298) -> (x-y=w10297:dbl)
                                n9852 = Absolute Value(x=w10297) -> (abs(x)=w10296:dbl)
                                n9853 = Multiply(x=w10296, y=w10295) -> (x*y=w10294:dbl)
                                n9854 = Divide(x=w10294, y=24000.0) -> (x/y=w10291:dbl)
                                n9855 = Subtract(x=w10291, y=w10292) -> (x-y=w10290:dbl)
                                n9856 = Absolute Value(x=w10290) -> (abs(x)=w10289:dbl)
                                }
                                }
                                n9857 = local write "Buffer-C Volume\nleft to be Pumped"(w10276) -> ()
                                }
                                frame #2 {
                                n9858 = local read "Buffer-C2 Dispense\nFlow Rate (ul/min)"() -> (w10308:dbl)
                                n9859 = local read "Buffer-C2 Pumping\nResolution"() -> (w10307:T2)
                                n9860 = local read "VISA Refnum in\nfor Pump"() -> (w10310:refnum<visa-resource-name>)
                                n9861 = local read "Volume of Syringe"() -> (w10309:dbl)
                                n9862 = call "GoToAbsolutePosition(SubVI).vi"("Absolute Volume Position in Syringe (in ul)"=0.0, "Volume of Syringe"=w10309, "Resolution of Pumping"=w10307, "Flow Rate (ul/min)"=w10308, "VISA Refnum in"=w10310) -> ()  [unwired: 6 in, 1 out]
                                n9863 = local write "External Valve \nOpen"(FALSE ("External Valve \nOpen")) -> ()
                                n9864 = local write "Valve V3 Open"(TRUE ("Valve V3 Open")) -> ()
                                n9865 = local write "Valve V7 Open"(FALSE ("Valve V3 Open")) -> ()
                                n9866 = local write "Valve V5 Open"(TRUE ("Valve V1 Open")) -> ()
                                n9867 = local write "Valve V6 Open"(TRUE ("Valve V2 Open")) -> ()
                                n9868 = local write "Valve V4 Open"(TRUE ("Valve V4 Open")) -> ()
                                }
                                frame #3 {
                                n9869 = local read "Buffer-C2 Pumping\nResolution"() -> (w10316:T2)
                                n9870 = local read "Initial Plunger Position"() -> (w10315:dbl)
                                n9871 = local read "VISA Refnum in\nfor Pump"() -> (w10317:refnum<visa-resource-name>)
                                n9872 = local read "Position\nNow"() -> (w10313:dbl)
                                n9873 = local read "Volume of Syringe"() -> (w10314:dbl)
                                n9874 = local write "Volume being Injected \nin this process"(0.0) -> ()
                                n9875 = local write "Pause Data Collection"(FALSE) -> ()
                                n9876 = while {
                                tunnel: w10317 -> [w10324]
                                tunnel: w10316 -> [w10323]
                                tunnel: w10315 -> [w10319]
                                tunnel: w10314 -> [w10322]
                                tunnel: w10313 -> [w10318]
                                stop <- w10320 stop-if-true
                                n9877 = stacked-sequence {
                                tunnel: w10324 -> [w10330 w10352 w10381]
                                tunnel: w10323 -> [w10329 w10351 _]
                                tunnel: w10319 -> [w10327 _ _]
                                tunnel: w10322 -> [w10326 w10349 _]
                                tunnel: [_ _ w10375] -> w10320
                                tunnel: w10318 -> [_ w10347 _]
                                frame #0 {
                                # "From here on 'True Volume being injected \nin this process' represents the true total \nvolume in this process"
                                n9878 = call "AbsolutePlungerPosition (SubVI).vi"("VISA Refnum in"=w10330) -> ("Plunger Position"=w10328:i32)  [unwired: 10 in]
                                n9879 = case shown="..\"Standard Pumping\"" w10329 {
                                tunnel: w10328 -> [w10338 w10346]
                                tunnel: w10327 -> [w10337 w10345]
                                tunnel: w10326 -> [w10334 w10342]
                                tunnel: [w10331 w10339] -> w10325
                                frame .."Standard Pumping" {
                                n9880 = Subtract(x=w10338, y=w10337) -> (x-y=w10336:dbl)
                                n9881 = Absolute Value(x=w10336) -> (abs(x)=w10335:dbl)
                                n9882 = Multiply(x=w10335, y=w10334) -> (x*y=w10333:dbl)
                                n9883 = Divide(x=w10333, y=3000.0) -> (x/y=w10331:dbl)
                                }
                                frame "High Resolution Pumping".. {
                                n9884 = Subtract(x=w10346, y=w10345) -> (x-y=w10344:dbl)
                                n9885 = Absolute Value(x=w10344) -> (abs(x)=w10343:dbl)
                                n9886 = Multiply(x=w10343, y=w10342) -> (x*y=w10341:dbl)
                                n9887 = Divide(x=w10341, y=24000.0) -> (x/y=w10339:dbl)
                                }
                                }
                                n9888 = local write "True Volume being \ninjected in this\nprocess"(w10325) -> ()
                                }
                                frame #1 {
                                # "From here on 'Volume being injected \nin this process' represents the volume \nin this sub process"
                                n9889 = call "AbsolutePlungerPosition (SubVI).vi"("VISA Refnum in"=w10352) -> ("Plunger Position"=w10350:i32)  [unwired: 10 in]
                                n9890 = case shown="\"High Resolution Pumping\".." w10351 {
                                tunnel: w10350 -> [w10360 w10368]
                                tunnel: w10347 -> [w10359 w10367]
                                tunnel: w10349 -> [w10356 w10364]
                                tunnel: [w10353 w10361] -> w10348
                                frame .."Standard Pumping" {
                                n9891 = Subtract(x=w10360, y=w10359) -> (x-y=w10358:dbl)
                                n9892 = Absolute Value(x=w10358) -> (abs(x)=w10357:dbl)
                                n9893 = Multiply(x=w10357, y=w10356) -> (x*y=w10355:dbl)
                                n9894 = Divide(x=w10355, y=3000.0) -> (x/y=w10353:dbl)
                                }
                                frame "High Resolution Pumping".. {
                                n9895 = Subtract(x=w10368, y=w10367) -> (x-y=w10366:dbl)
                                n9896 = Absolute Value(x=w10366) -> (abs(x)=w10365:dbl)
                                n9897 = Multiply(x=w10365, y=w10364) -> (x*y=w10363:dbl)
                                n9898 = Divide(x=w10363, y=24000.0) -> (x/y=w10361:dbl)
                                }
                                }
                                n9899 = local write "Volume being Injected \nin this process"(w10348) -> ()
                                }
                                frame #2 {
                                n9900 = local read "Capillary purge \nvolume after every\ngrid plunging"() -> (w10370:dbl)
                                n9901 = local read "Stop for End of \nExperiment \nand Data Writing"() -> (w10374:bool)
                                n9902 = local read "Volume being Injected \nin this process"() -> (w10371:dbl)
                                n9903 = local read "Re-SEC"() -> (w10373:bool)
                                n9904 = call "AbsolutePlungerPositionStatus (SubVI).vi"("VISA Refnum in"=w10381) -> ("read buffer"=w10380:string)  [unwired: 10 in]
                                n9905 = call <vilib>:"Trim Whitespace.vi"("string"=w10380) -> ("trimmed string"=w10379:string)  [unwired: 1 in]
                                n9906 = Greater Or Equal?(x=w10371, y=w10370) -> (x >= y?=w10369:bool)
                                n9907 = Equal?(x=w10379, y="/0`\u0003") -> (x = y?=w10377:bool)
                                n9908 = Or(x=w10374, y=w10373) -> (x .or. y?=w10372:bool)
                                n9909 = Or(x=w10369, y=w10372) -> (x .or. y?=w10376:bool)
                                n9910 = Or(x=w10377, y=w10376) -> (x .or. y?=w10375:bool)
                                }
                                }
                                n9911 = Wait (ms)(milliseconds to wait=u32 100) -> ()  [unwired: 1 out]
                                }
                                }
                                frame #4 {
                                n9912 = local read "VISA Refnum in\nfor Pump"() -> (w10382:refnum<visa-resource-name>)
                                n9913 = call "HardStopCurrentProcess (SubVI).vi"("VISA Refnum in"=w10382) -> ()  [unwired: 11 in]
                                }
                                }
                                }
                                }
                                }
                                frame #4 {
                                n9914 = local write "Valve V3 Open"(FALSE ("Valve V3 Open")) -> ()
                                n9915 = local write "Valve V7 Open"(FALSE ("Valve V3 Open")) -> ()
                                n9916 = local write "Valve V5 Open"(FALSE ("Valve V1 Open")) -> ()
                                n9917 = local write "Valve V6 Open"(FALSE ("Valve V2 Open")) -> ()
                                n9918 = local write "Valve V4 Open"(FALSE ("Valve V4 Open")) -> ()
                                }
                                frame #5 {
                                n9919 = while {
                                stop <- w10392 stop-if-true
                                n9920 = local read "Stop for End of \nExperiment \nand Data Writing"() -> (w10390:bool)
                                n9921 = local read "Re-deposit Sample\nonto Grid"() -> (w10393:bool)
                                n9922 = local read "Re-SEC"() -> (w10391:bool)
                                n9923 = Or(x=w10390, y=w10391) -> (x .or. y?=w10389:bool)
                                n9924 = Or(x=w10393, y=w10389) -> (x .or. y?=w10392:bool)
                                }
                                n9925 = One Button Dialog(message="Do you want to deposit sample on another grid? If yes, turn on 'Re-deposit Sample onto Grid'. Else turn on Re-SEC to do SEC again or STOP to end the experiment") -> ()  [unwired: 1 in, 1 out]
                                }
                                frame #6 {
                                n9926 = local write "Valve V4 Open"(TRUE ("Valve V4 Open")) -> ()
                                n9927 = local write "Valve V3 Open"(TRUE ("Valve V3 Open")) -> ()
                                n9928 = local write "Valve V7 Open"(FALSE ("Valve V3 Open")) -> ()
                                n9929 = local write "Valve V5 Open"(TRUE ("Valve V1 Open")) -> ()
                                n9930 = local write "Valve V6 Open"(TRUE ("Valve V2 Open")) -> ()
                                }
                                frame #7 {
                                n9931 = local read "Re-deposit Sample\nonto Grid"() -> (w10399:bool)
                                n9932 = case shown="True" w10399 {
                                frame False {
                                n9933 = local write "Suction On/Off"(FALSE ("Suction On/Off")) -> ()
                                }
                                frame True {
                                n9934 = stacked-sequence {
                                frame #0 {
                                n9935 = local read "VISA Refnum in\nfor Pump"() -> (w10402:refnum<visa-resource-name>)
                                n9936 = call "AbsolutePlungerPosition (SubVI).vi"("VISA Refnum in"=w10402) -> ("Plunger Position"=w10401:i32)  [unwired: 10 in]
                                n9937 = local write "Position\nNow"(w10401) -> ()
                                }
                                frame #1 {
                                n9938 = local read "Buffer-C2 Pumping\nResolution"() -> (w10404:T2)
                                n9939 = case shown="\"Standard Pumping\", Default" w10404 {
                                tunnel: [w10405 w10416] -> w10403
                                frame "Standard Pumping", Default {
                                n9940 = local read "Buffer-C2 Volume \nto be Pumped"() -> (w10408:dbl)
                                n9941 = local read "Volume of Syringe"() -> (w10411:dbl)
                                n9942 = local read "Initial Plunger Position"() -> (w10415:dbl)
                                n9943 = local read "Position\nNow"() -> (w10414:dbl)
                                n9944 = Subtract(x=w10415, y=w10414) -> (x-y=w10413:dbl)
                                n9945 = Absolute Value(x=w10413) -> (abs(x)=w10412:dbl)
                                n9946 = Multiply(x=w10412, y=w10411) -> (x*y=w10410:dbl)
                                n9947 = Divide(x=w10410, y=3000.0) -> (x/y=w10407:dbl)
                                n9948 = Subtract(x=w10407, y=w10408) -> (x-y=w10406:dbl)
                                n9949 = Absolute Value(x=w10406) -> (abs(x)=w10405:dbl)
                                }
                                frame "High Resolution Pumping" {
                                n9950 = local read "Buffer-C2 Volume \nto be Pumped"() -> (w10419:dbl)
                                n9951 = local read "Volume of Syringe"() -> (w10422:dbl)
                                n9952 = local read "Initial Plunger Position"() -> (w10426:dbl)
                                n9953 = local read "Position\nNow"() -> (w10425:dbl)
                                n9954 = Subtract(x=w10426, y=w10425) -> (x-y=w10424:dbl)
                                n9955 = Absolute Value(x=w10424) -> (abs(x)=w10423:dbl)
                                n9956 = Multiply(x=w10423, y=w10422) -> (x*y=w10421:dbl)
                                n9957 = Divide(x=w10421, y=24000.0) -> (x/y=w10418:dbl)
                                n9958 = Subtract(x=w10418, y=w10419) -> (x-y=w10417:dbl)
                                n9959 = Absolute Value(x=w10417) -> (abs(x)=w10416:dbl)
                                }
                                }
                                n9960 = local write "Buffer-C Volume\nleft to be Pumped"(w10403) -> ()
                                }
                                frame #2 {
                                n9961 = local read "Buffer-C2 Dispense\nFlow Rate (ul/min)"() -> (w10430:dbl)
                                n9962 = local read "Buffer-C2 Pumping\nResolution"() -> (w10429:T2)
                                n9963 = local read "VISA Refnum in\nfor Pump"() -> (w10432:refnum<visa-resource-name>)
                                n9964 = local read "Volume of Syringe"() -> (w10431:dbl)
                                n9965 = call "GoToAbsolutePosition(SubVI).vi"("Absolute Volume Position in Syringe (in ul)"=0.0, "Volume of Syringe"=w10431, "Resolution of Pumping"=w10429, "Flow Rate (ul/min)"=w10430, "VISA Refnum in"=w10432) -> ()  [unwired: 6 in, 1 out]
                                n9966 = local write "Suction On/Off"(FALSE ("Suction On/Off")) -> ()
                                }
                                }
                                }
                                }
                                }
                                frame #8 {
                                n9967 = local read "Stop for End of \nExperiment \nand Data Writing"() -> (w10434:bool)
                                n9968 = local read "Re-SEC"() -> (w10435:bool)
                                n9969 = Or(x=w10434, y=w10435) -> (x .or. y?=w10433:bool)
                                n9970 = case shown="True" w10433 {
                                frame False {
                                }
                                frame True {
                                n9971 = local read "VISA Refnum in\nfor Pump"() -> (w10436:refnum<visa-resource-name>)
                                n9972 = call "HardStopCurrentProcess (SubVI).vi"("VISA Refnum in"=w10436) -> ()  [unwired: 11 in]
                                }
                                }
                                }
                                }
                                }
                                }
                                n9973 = local read "Stop for End of \nExperiment \nand Data Writing"() -> (w10172:bool)
                                n9974 = local read "Divert Sample \nonto Grid"() -> (w10175:bool)
                                n9975 = local read "Re-SEC"() -> (w10173:bool)
                                n9976 = Not(x=w10175) -> (.not. x?=w10174:bool)
                                n9977 = Or(x=w10172, y=w10173) -> (x .or. y?=w10171:bool)
                                n9978 = Or(x=w10174, y=w10171) -> (x .or. y?=w10176:bool)
                                }
                              }
                            }
                            n9979 = local write "Discard fluid \nprior to 1st \ndeposition"(TRUE ("Discard fluid \nprior to 1st \ndeposition")) -> ()
                          }
                        }
                      }
                      frame #17 {
                        n9980 = local read "Stopper that ends \nthe main loops"() -> (w10438:bool)
                        n9981 = local read "Re-SEC"() -> (w10439:bool)
                        n9982 = Wait (ms)(milliseconds to wait=u32 500) -> ()  [unwired: 1 out]
                        n9983 = Or(x=w10438, y=w10439) -> (x .or. y?=w10437:bool)
                        n9984 = case shown="True" w10437 {
                          frame False {
                          }
                          frame True {
                            n9985 = local read "VISA Refnum in\nfor Pump"() -> (w10444:refnum<visa-resource-name>)
                            n9986 = call "HardStopCurrentProcess (SubVI).vi"("VISA Refnum in"=w10444) -> ()  [unwired: 11 in]
                          }
                        }
                        n9987 = local write "Divert Sample \nonto Grid"(FALSE ("Divert Sample \nonto Grid")) -> ()
                        n9988 = local write "Pause Data Collection"(TRUE ("Pause Data Collection")) -> ()
                        n9989 = local write "Start the Process"(FALSE ("Start the Process")) -> ()
                      }
                      frame #18 {
                        n9990 = local read "Stop for End of \nExperiment \nand Data Writing"() -> (w10451:bool)
                        n9991 = local read "Start the Process"() -> (w10450:bool)
                        n9992 = Or(x=w10450, y=w10451) -> (x .or. y?=w10449:bool)
                        n9993 = case shown="False" w10449 {
                          frame False {
                            n9994 = while {
                              stop <- w10457 stop-if-true
                              n9995 = local read "Stop for End of \nExperiment \nand Data Writing"() -> (w10459:bool)
                              n9996 = local read "Start the Process"() -> (w10458:bool)
                              n9997 = Or(x=w10458, y=w10459) -> (x .or. y?=w10457:bool)
                              n9998 = Wait (ms)(milliseconds to wait=u32 100) -> ()  [unwired: 1 out]
                            }
                            n9999 = One Button Dialog(message="Do you want to re-introduce sample into column-2 and elute? If yes, adjust the re-introduction volume into column-2 and elution parameters for column-2 and turn on the 'Start the Process' button . If no, turn on the 'Stop for End of Experiment and Data Writing'.") -> ()  [unwired: 1 in, 1 out]
                          }
                          frame True {
                            n10000 = local read "Stop for End of \nExperiment \nand Data Writing"() -> (w10460:bool)
                            n10001 = case shown="True" w10460 {
                              frame False {
                              }
                              frame True {
                                n10002 = local write "Valve V1 Open"(FALSE ("Valve V1 Open")) -> ()
                                n10003 = local write "Valve V2 Open"(FALSE ("Valve V2 Open")) -> ()
                                n10004 = local write "Valve V4 Open"(FALSE ("Valve V4 Open")) -> ()
                                n10005 = local write "Valve V3 Open"(FALSE ("Valve V3 Open")) -> ()
                                n10006 = local write "Valve V5 Open"(FALSE ("Valve V5 Open")) -> ()
                                n10007 = local write "Valve V6 Open"(FALSE ("Valve V6 Open")) -> ()
                                n10008 = local write "Valve V7 Open"(FALSE ("Valve V7 Open")) -> ()
                              }
                            }
                          }
                        }
                        n10009 = local write "Sample Volume Diverted\ninto Column-2"(0.0 ("Sample Volume Diverted\ninto Column-2")) -> ()
                        n10010 = local write "Buffer-C Volume\nleft to be Pumped"(0.0 ("Buffer-C Volume\nleft to be Pumped")) -> ()
                        n10011 = local write "Vol_previous"(0.0 ("Vol_previous")) -> ()
                        n10012 = local write "Vol_now"(0.0 ("Vol_now")) -> ()
                        n10013 = local write "Elution of Column-2"(FALSE ("Elution of Column-2")) -> ()
                        n10014 = local write "SEC On"(FALSE ("SEC On")) -> ()
                        n10015 = local write "Volume being Injected \nin this process"(0.0 ("Volume being Injected \nin this process")) -> ()
                      }
                    }
                  }
                }
              }
              frame True {
                n10016 = local write "Pause Data Collection"(FALSE ("Pause Data Collection")) -> ()
              }
            }
          }
        }
        n10017 = local read "Stop for End of \nExperiment \nand Data Writing"() -> (w527:bool)
        n10018 = local write "Stopper that ends \nthe main loops"(w527) -> ()
        n10019 = local read "Stopper that ends \nthe main loops"() -> (w528:bool)
      }
      n10020 = invoke class="KCubeInertialMotorControl" method="CreateDevice"(reference=w74, error in=w81) -> (reference out=w76:refnum<k24>, error out=w75:errorcluster)  [unwired: 1 in, 1 out]
      n10021 = property class="KCubeInertialMotorControl"(reference=w76, error in=w75) -> (reference out=w85:refnum<k24>, error out=w79:errorcluster, "Device"=w77:refnum<k24>)
      n10022 = while {
        tunnel: w77 -> [w111]
        tunnel: [w109] -> w78
        tunnel: w79 -> [w107]
        tunnel: [w106] -> w80
        stop <- w110 stop-if-true
        n10023 = invoke class="KCubeInertialMotor" method="IsSettingsInitialized"(reference=w111, error in=w107) -> (reference out=w109:refnum<k24>, error out=w106:errorcluster, "IsSettingsInitialized"=w110:bool)  [unwired: 1 in]
        n10024 = Wait (ms)(milliseconds to wait=u32 50) -> ()  [unwired: 1 out]
      }
      n10025 = Get Date/Time In Seconds() -> (seconds since 1Jan1904=w37:timestamp)
      n10026 = Get Date/Time In Seconds() -> (seconds since 1Jan1904=w34:timestamp)
      n10027 = Get Date/Time In Seconds() -> (seconds since 1Jan1904=w46:timestamp)
      n10028 = Get Date/Time In Seconds() -> (seconds since 1Jan1904=w43:timestamp)
      n10029 = Get Date/Time In Seconds() -> (seconds since 1Jan1904=w54:timestamp)
      n10030 = Get Date/Time In Seconds() -> (seconds since 1Jan1904=w51:timestamp)
      n10031 = Get Date/Time In Seconds() -> (seconds since 1Jan1904=w95:timestamp)
      n10032 = Get Date/Time In Seconds() -> (seconds since 1Jan1904=w91:timestamp)
      n10033 = Get Date/Time In Seconds() -> (seconds since 1Jan1904=w67:timestamp)
      n10034 = Bundle By Name("Y"=dbl[] [], "t0"=w34, "dt"=0.001) -> (w32:waveform(dbl))  [unwired: 1 in]
      n10035 = Bundle By Name("Y"=dbl[] [], "t0"=w37, "dt"=0.001) -> (w33:waveform(dbl))  [unwired: 1 in]
      n10036 = Bundle By Name("Y"=dbl[] [], "t0"=w43, "dt"=0.001) -> (w41:waveform(dbl))  [unwired: 1 in]
      n10037 = Bundle By Name("Y"=dbl[] [], "t0"=w46, "dt"=0.001) -> (w42:waveform(dbl))  [unwired: 1 in]
      n10038 = Bundle By Name("Y"=dbl[] [], "t0"=w51, "dt"=0.001) -> (w49:waveform(dbl))  [unwired: 1 in]
      n10039 = Bundle By Name("Y"=dbl[] [], "t0"=w54, "dt"=0.001) -> (w50:waveform(dbl))  [unwired: 1 in]
      n10040 = Bundle By Name("Y"=dbl[] [], "t0"=w91, "dt"=0.001) -> (w90:waveform(dbl))  [unwired: 1 in]
      n10041 = Bundle By Name("Y"=dbl[] [], "t0"=w95, "dt"=0.001) -> (w94:waveform(dbl))  [unwired: 1 in]
      n10042 = invoke class="KCubeInertialMotor" method="StartPolling"(reference=w78, error in=w80, "ms"=250) -> (reference out=w10:refnum<k24>, error out=w9:errorcluster)  [unwired: 1 in, 2 out]
      n10043 = Bundle By Name("Y"=dbl[] [], "t0"=w67, "dt"=0.1) -> (w72:waveform(dbl))  [unwired: 1 in]
      n10044 = while {
        shift-right: [w10496] -> w87
        shift-left: w94 -> [w10503]
        shift-right: [w10488] -> w88
        shift-left: w90 -> [w10489]
        shift-right: [w10483] -> _
        shift-left: w50 -> [w10484]
        shift-right: [w10481] -> _
        shift-left: w49 -> [w10482]
        shift-right: [w10478] -> _
        shift-left: w42 -> [w10480]
        shift-right: [w10477] -> _
        shift-left: w41 -> [w10479]
        shift-right: [w10472] -> _
        shift-left: w32 -> [w10474]
        shift-right: [w10473] -> _
        shift-left: w33 -> [w10475]
        stop <- w10491 stop-if-true
        # "Voltage applied in volts\nfor Opamps"
        # "Input Voltage Circuit  for the Amplifier"
        # "Amplified Signal in Volts"
        n10045 = local read "Stop for End of \nExperiment \nand Data Writing"() -> (w10487:bool)
        n10046 = local read "Volume being Injected \ntill the end of previous \nprocess"() -> (w10494:dbl)
        n10047 = local read "Pause Data Collection"() -> (w10493:bool)
        n10048 = local read "Affinity Elution \nis Approaching"() -> (w10476:bool)
        n10049 = local read "Affinity Elution On"() -> (w10469:bool)
        n10050 = local read "Volume being Injected \nin this process"() -> (w10495:dbl)
        n10051 = local read "SEC On"() -> (w10486:bool)
        n10052 = case shown="True" w10493 {
          frame False {
          }
          frame True {
            n10053 = local read "Volume being Injected \ntill the end of previous \nprocess"() -> (w10556:dbl)
            n10054 = while {
              stop <- w10558 continue-if-true
              n10055 = Wait (ms)(milliseconds to wait=u32 10) -> ()  [unwired: 1 out]
              n10056 = local read "Pause Data Collection"() -> (w10558:bool)
            }
            n10057 = local read "Volume being Injected \nin this process"() -> (w10554:dbl)
            n10058 = Add(x=w10554, y=w10556) -> (x+y=w10555:dbl)
            n10059 = local write "Volume being Injected \ntill the end of previous \nprocess"(w10555) -> ()
          }
        }
        n10060 = case shown="True" w10487 {
          frame False {
          }
          frame True {
            n10061 = stacked-sequence {
              frame #0 {
                n10062 = local write "Stopper that ends \nthe main loops"(TRUE) -> ()
                n10063 = local write "Start the Process"(TRUE) -> ()
                n10064 = local write "Pause Data Collection"(FALSE) -> ()
                n10065 = local write "Pause /Continue"(FALSE) -> ()
                n10066 = Wait (ms)(milliseconds to wait=250) -> ()  [unwired: 1 out]
              }
              frame #1 {
              }
            }
          }
        }
        n10067 = Add(x=w10494, y=w10495) -> (x+y=w10490:dbl)
        n10068 = call "Convert from Dynamic Data4"("Dynamic Data Type"=w10490) -> ("Waveform"=w10470:waveform(dbl))  [unwired: 3 in]
        n10069 = local write "Total Volume \nbeing Injected"(w10490) -> ()
        n10070 = call-poly <vilib>:"Append Waveforms.vi"("waveform B"=w10470, "waveform A"=w10489) -> ("waveform out"=w10488:waveform(dbl))  [unwired: 8 in, 1 out]
        n10071 = call "DAQ AO-0"("data"=-5) -> ()  [unwired: 17 in, 2 out]
        n10072 = call "Convert from Dynamic Data2"("Dynamic Data Type"=w10488) -> ("Array"=w10498:dbl[])  [unwired: 3 in]
        n10073 = local read "Stopper that ends \nthe main loops"() -> (w10491:bool)
        n10074 = call "DAQ Assistant"() -> ("data"=w10502:dynamicdata)  [unwired: 17 in, 2 out]
        n10075 = call "Convert from Dynamic Data"("Dynamic Data Type"=w10502) -> ("Waveform"=w10501:waveform(dbl))  [unwired: 3 in]
        n10076 = Multiply(x=-1, y=w10501) -> (x*y=w10471:waveform(dbl))
        n10077 = case shown="True" w10486 {
          tunnel: w10484 -> [w10539 w10546]
          tunnel: w10471 -> [_ w10545]
          tunnel: [w10538 w10544] -> w10483
          tunnel: w10482 -> [w10537 w10542]
          tunnel: [w10536 w10540] -> w10481
          tunnel: w10470 -> [_ w10541]
          frame False {
            n10078 = call-poly <vilib>:"Append Waveforms.vi"("waveform B"=waveform(dbl) {"t0"=timestamp(0 s since 1904-01-01), "dt"=1.0, "Y"=[]}, "waveform A"=w10537) -> ("waveform out"=w10536:waveform(dbl))  [unwired: 8 in, 1 out]
            n10079 = call-poly <vilib>:"Append Waveforms.vi"("waveform B"=waveform(dbl) {"t0"=timestamp(0 s since 1904-01-01), "dt"=1.0, "Y"=[]}, "waveform A"=w10539) -> ("waveform out"=w10538:waveform(dbl))  [unwired: 8 in, 1 out]
          }
          frame True {
            n10080 = call-poly <vilib>:"Append Waveforms.vi"("waveform B"=w10541, "waveform A"=w10542) -> ("waveform out"=w10540:waveform(dbl))  [unwired: 8 in, 1 out]
